vi "Problem3.6.vi"() -> ()   [LabVIEW 2019]
panel:
  in  "RobotAction":bool
  out "Robot Action":bool
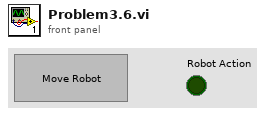
[diagram p1: front panel]
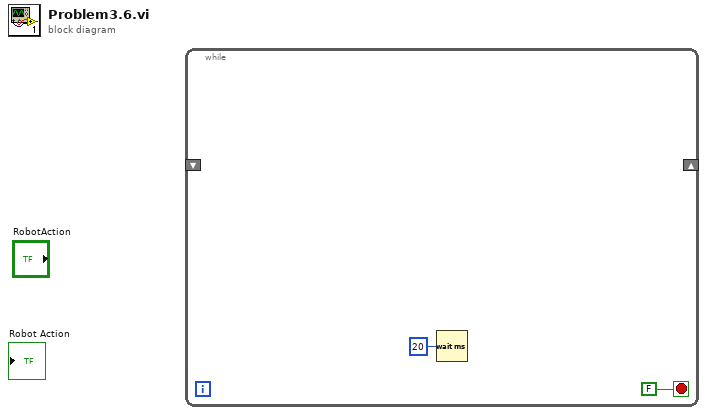
[diagram p0: block diagram]
diagram:
  n1 = while {
    shift-right: _ -> [_]
    shift-left: _ -> [_]
    stop <- FALSE stop-if-true
    n2 = Wait (ms)(milliseconds to wait=u32 20) -> ()  [unwired: 1 out]
  }
